vi "XIPIN_G.709_FEC_Encoder_Decoder_1_0.vi"   [LabVIEW 2017]
doc: "The G.709 FEC LogiCore is a high speed, compact module that implements the ITU G.709 Forward Error Correction as specified in Annex A of the standard.\n------------------------------------\n<b>Need License</b> : Yes\n<b>Interface</b> : AXI4-Stream"
uses:
  <vilib>/rvi/XilinxIP/XIPIN_XNode/niFpgaXIPIN.xnode
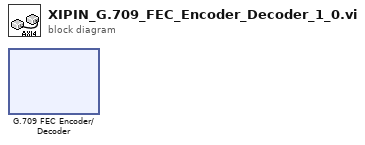
[diagram p0: block diagram]
diagram:
  n1 = xnode ("G.709 FEC Encoder/Decoder")() -> ()
